vi "UIRef.vi"(8 "error in":errorcluster, 11 "EngineTags in":refnum<class "EngineTags.lvclass">) -> (0 "error out":errorcluster, 2 "VI refnum":refnum<vi>, 3 "EngineTags out":refnum<class "EngineTags.lvclass">)   [LabVIEW 2013, in "PL Framework Configuration Tool.lvlib" / "EngineTags.lvclass"]
uses:
  EngineTags.lvclass
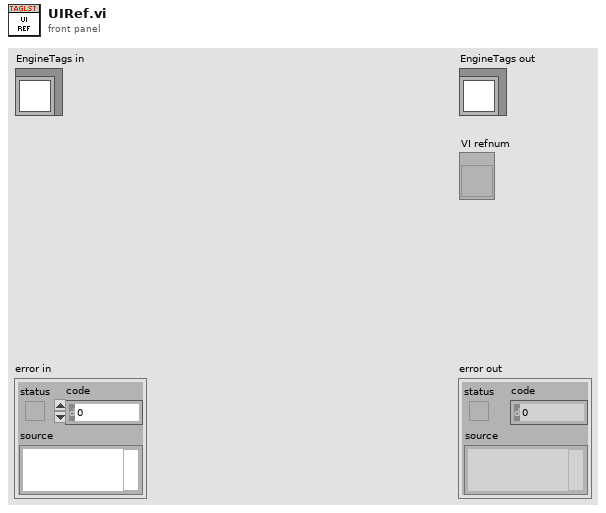
[diagram p1: front panel]
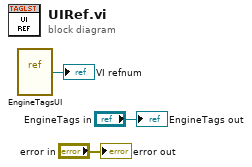
[diagram p0: block diagram]
diagram:
  n1 = vi-ref "EngineTagsUI.vi"() -> (→"VI refnum":refnum<vi>)
  "error out" <- "error in"
  "EngineTags out" <- "EngineTags in"
